vi "Read Strings And Values [].vi"(9 "Combobox in":refnum<class "Combobox.lvclass">) -> (3 "Combobox out":refnum<class "Combobox.lvclass">, 4 "Strings And Values []":T1)   [LabVIEW 2014, in "Raspberry Pi Compatible Compiler for LabVIEW.lvlib" / "Combobox.lvclass"]
uses:
  Combobox.lvclass
  <vilib>/Utility/miscctls.llb/LVComboBoxStrsAndValuesArrayTypeDef.ctl
  Combobox.lvclass/Combobox.ctl
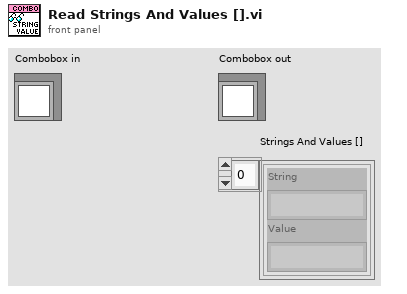
[diagram p1: front panel]
types:
  T1 = typedef "LVComboBoxStrsAndValuesArrayTypeDef.ctl" = cluster{"String":string, "Value":string}[]
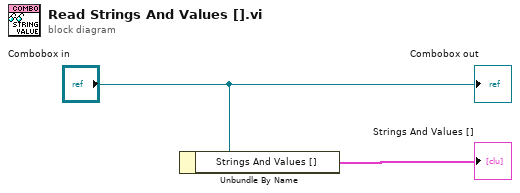
[diagram p0: block diagram]
diagram:
  n1 = Unbundle By Name("Combobox in") -> ("Strings And Values []"=→"Strings And Values []":T1)
  "Combobox out" <- "Combobox in"
